vi "Get Subchannel IDs.vi"(8 "error in":errorcluster, 11 "EventMessengerMData in":refnum<class "EventMessengerMData.lvclass">) -> (0 "error out":errorcluster, 2 "Subchannel IDs":string[](array[string]), 3 "EventMessengerMData out":refnum<class "EventMessengerMData.lvclass">)   [LabVIEW 2020, in "Event MessengerM.lvlib" / "EventMessengerMData.lvclass"]
uses:
  EventMessengerMData.lvclass
  EventMessengerMData.lvclass/EventMessengerMData.ctl
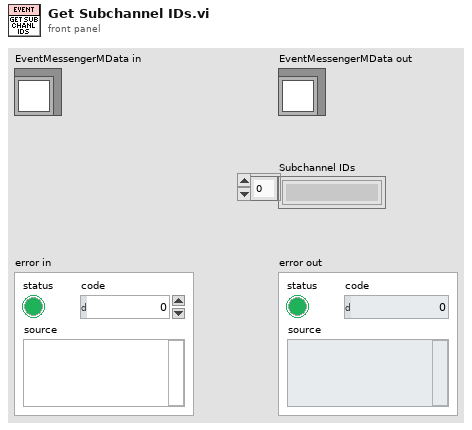
[diagram p1: front panel]
types:
  T1 = map{string, cluster{"Write Count":u32, "Reg Refnum":u32, "aborted?":bool, "last msg?":bool, "Event Refnum":refnum<user-event>}}
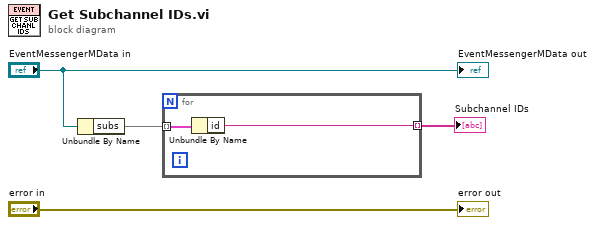
[diagram p0: block diagram]
diagram:
  n1 = Unbundle By Name("EventMessengerMData in") -> ("subs"=w2:T1)
  n2 = for {
    tunnel: w2 -> [w6] mode=indexing
    tunnel: [w5] -> w1 mode=indexing
    n3 = Unbundle By Name(w6) -> ("id"=w5:string)
  }
  "Subchannel IDs" <- w1
  "EventMessengerMData out" <- "EventMessengerMData in"
  "error out" <- "error in"
